vi "sub_makeGuess.vi"(9 "Array":T1[][](array[typedef]), 11 "Queue in":refnum<queue>) -> (1 "guess":T2, 3 "queue out":refnum<queue>)   [LabVIEW 2018]
uses:
  guess.ctl
  cell.ctl
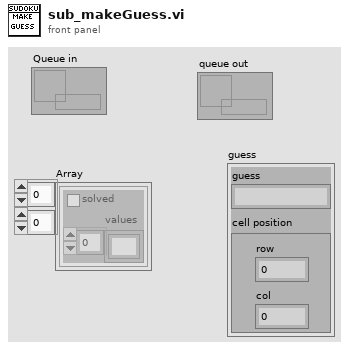
[diagram p1: front panel]
types:
  T1 = typedef "cell.ctl" = cluster{"solved":bool, "values":string[]}
  T2 = typedef "guess.ctl" = cluster{"cell position":cluster{"row":i32, "col":i32}, "guess":string}
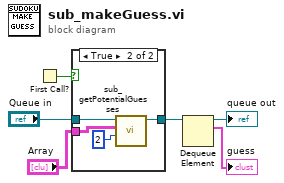
[diagram p0: block diagram]
diagram:
  n1 = First Call?() -> (First Call?: T/F=w2:bool)
  n2 = case shown="True" w2 {
    tunnel: "Array" -> [_ w11]
    tunnel: [w7 w10] -> w4
    tunnel: "Queue in" -> [w7 w8]
    frame False {
    }
    frame True {
      n3 = call "sub_getPotentialGuesses.vi"("# of potential options for the cell"=2, "solver array"=w11, "guess queue (in)"=w8) -> ("guess queue (out)"=w10:refnum<queue>)  [unwired: 8 in]
    }
  }
  n4 = Dequeue Element(queue=w4) -> (queue out=→"queue out":refnum<queue>, element=→"guess":T2)  [unwired: 2 in, 2 out]
